vi "tale of three indices.vi"(7 "selector":T2, 11 "tale of three indices -- int -- control":T1={"left"=0, "center"=0, "right"=0, "right most"=0, "left most"=0, "window"=0, "max win factor"=2, "max win"=2, "min win"=2}) -> (0 "no success ?":bool, 1 "at right end?":bool, 3 "tale of three indices -- int -- control out":T1={"left"=0, "center"=0, "right"=0, "right most"=0, "left most"=0, "window"=0, "max win factor"=2, "max win"=2, "min win"=2}, 5 "selector out":T2)   [LabVIEW 2018]
uses:
  tale of three indices -- int -- control.ctl
  tale of three indices -- selector -- control.ctl
  stack action -- control.ctl
  tale of three indices --state.ctl
  Q - not nan -- integer.vi
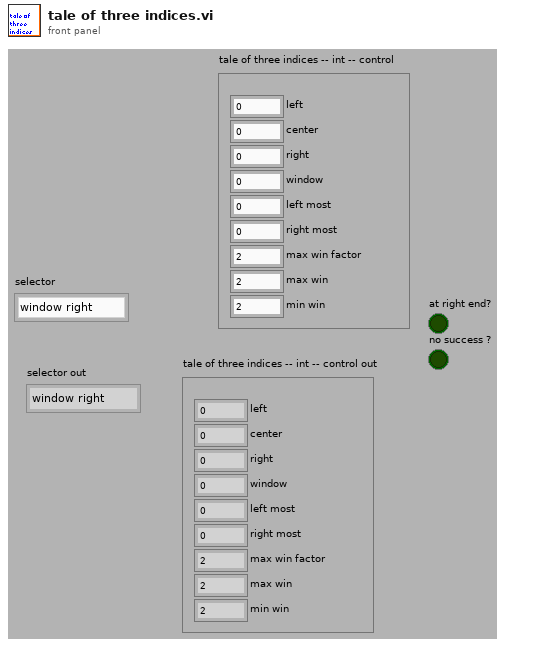
[diagram p1: front panel]
types:
  T1 = typedef "tale of three indices -- int -- control.ctl" = cluster{"left":i32, "center":i32, "right":i32, "right most":i32, "left most":i32, "window":i32, "max win factor":i32, "max win":i32, "min win":i32}
  T2 = typedef "tale of three indices -- selector -- control.ctl" = enum16{"window right", "window left", "balance", "shrink", "grow", "do nothing", "reset", "center right", "center left", "all left", "all right", "right wing shrink", "left wing shrink", "left wing grow", "right wing grow", "skew left", "skew right", "check"}
  T3 = typedef "stack action -- control.ctl" = enum16{"push", "pop", "check", "init"}
  T4 = typedef "tale of three indices --state.ctl" = enum16{"OK", "window stuck at left", "window stuck at right", "left wing shrink - able", "right wing shrink- able", "left wing broaden - able", "window right - able", "right wing broaden - able", "window left - able", "broaden - able", "shrink - able", "center right - able", "center left - able", "balance state"}
  T5 = enum16{"not a number", "above", "in range", "below"}
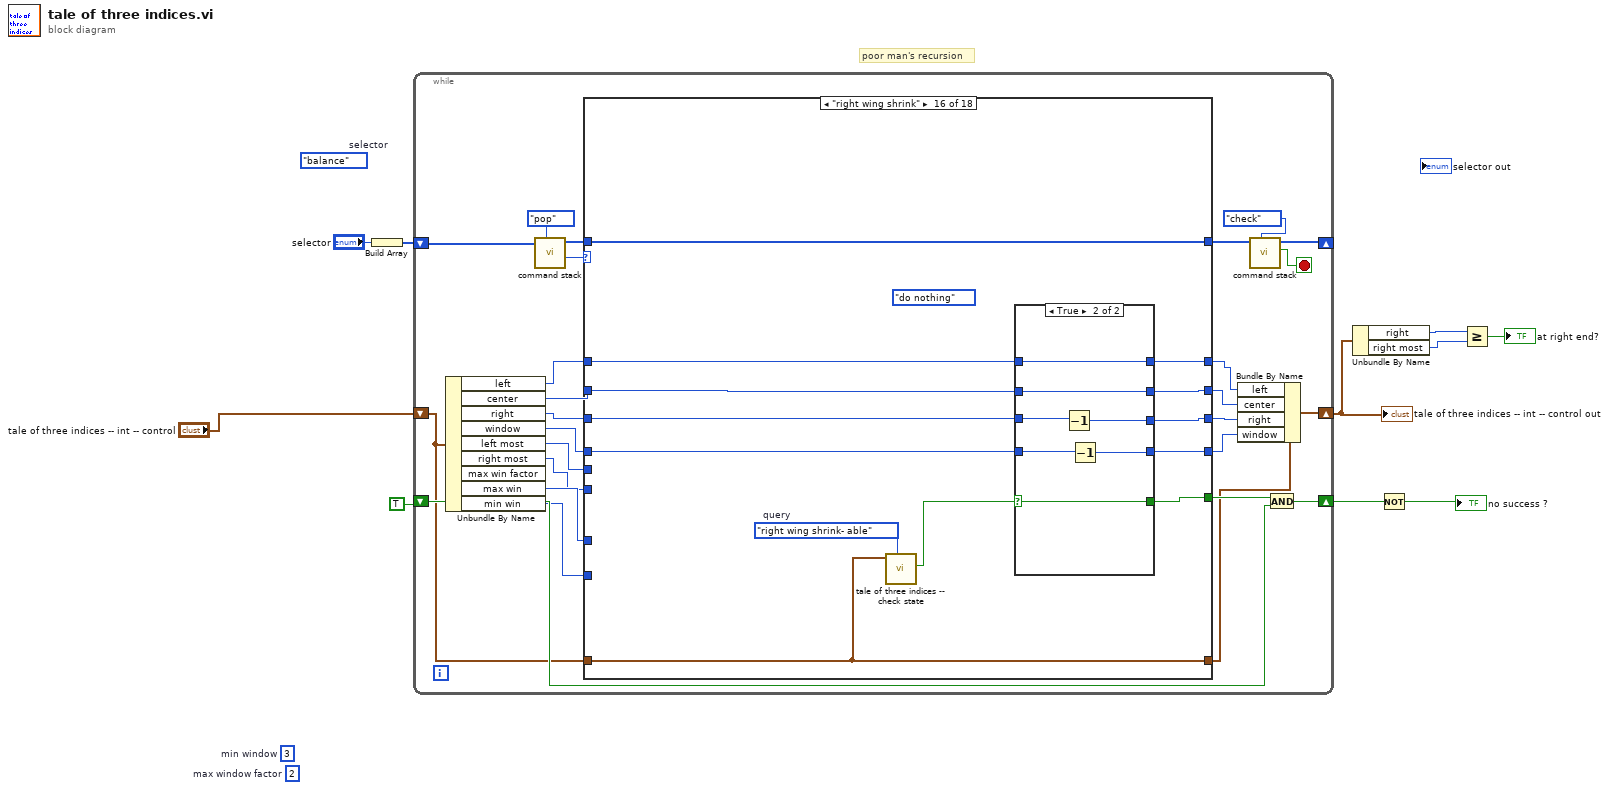
[diagram p0: block diagram]
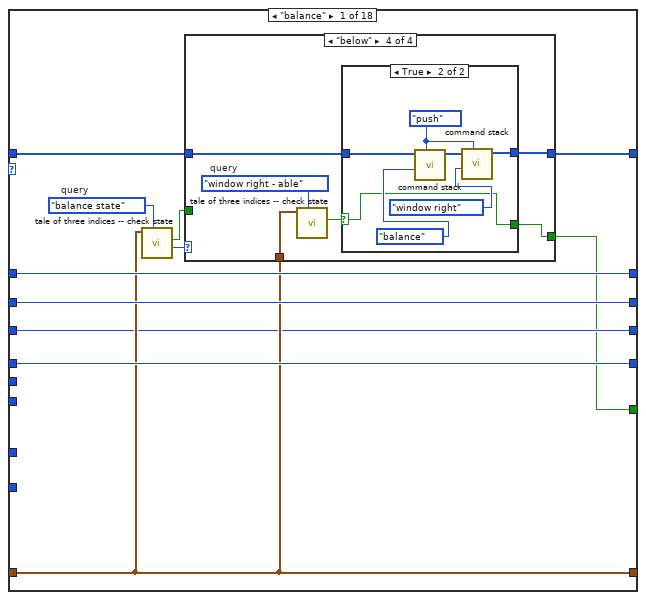
[diagram p2: hidden frame]
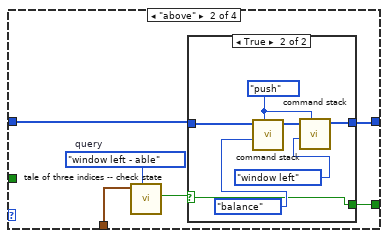
[diagram p4: hidden frame]
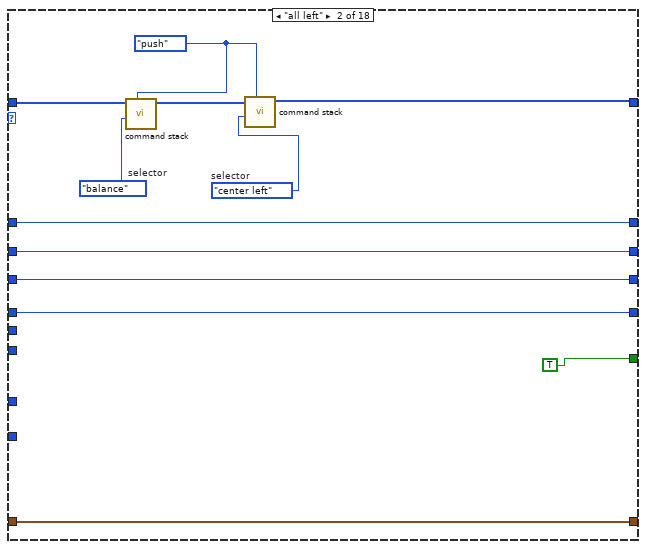
[diagram p8: hidden frame]
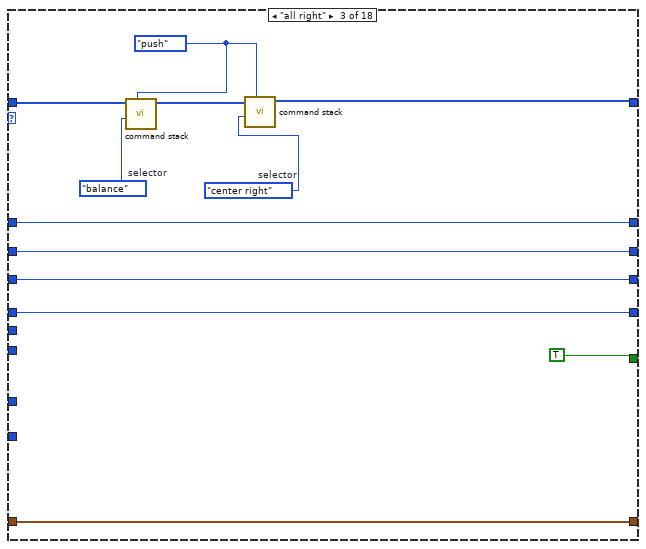
[diagram p9: hidden frame]
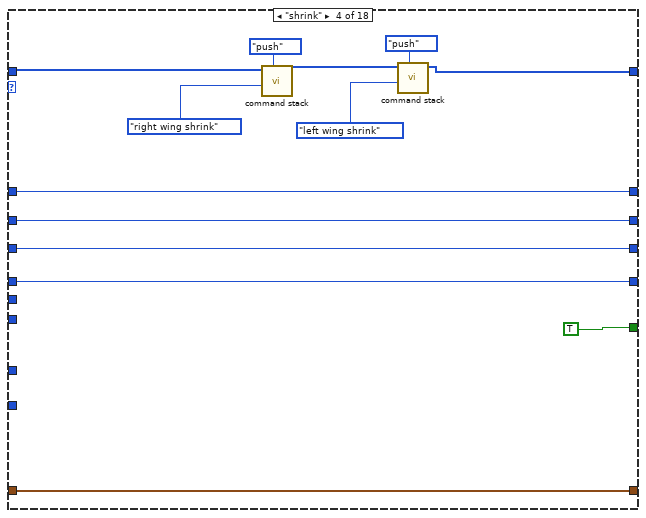
[diagram p10: hidden frame]
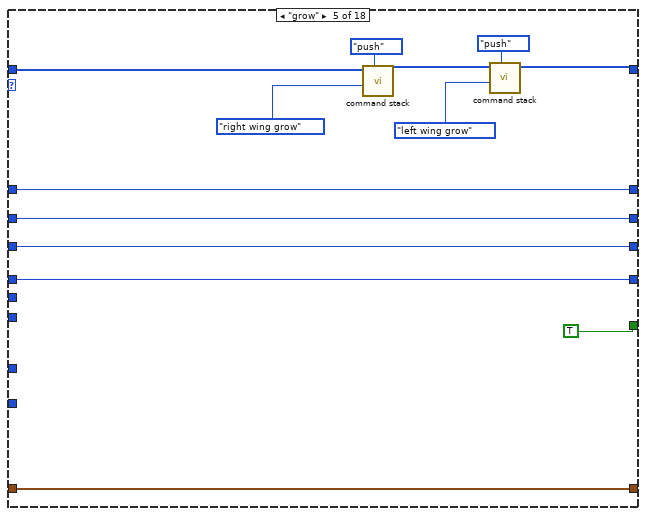
[diagram p11: hidden frame]
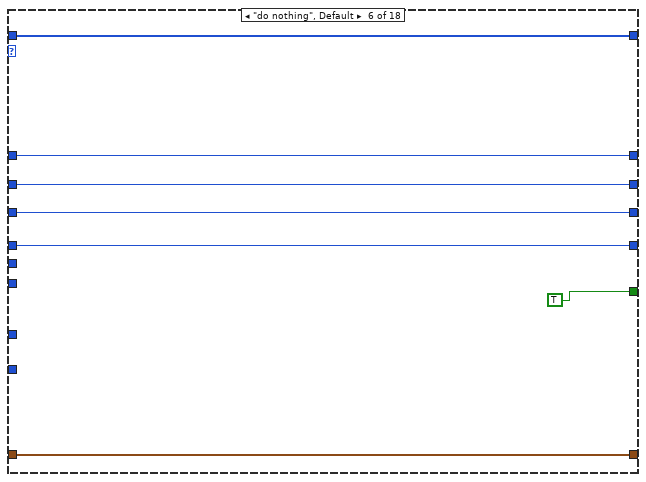
[diagram p12: hidden frame]
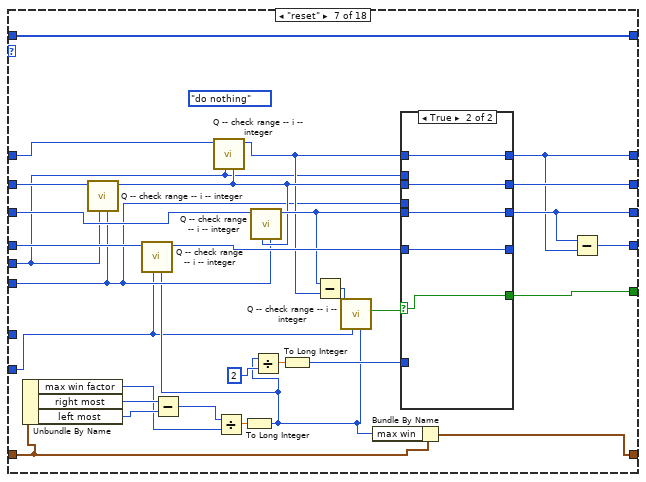
[diagram p13: hidden frame]
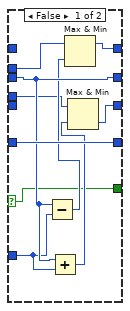
[diagram p14: hidden frame]
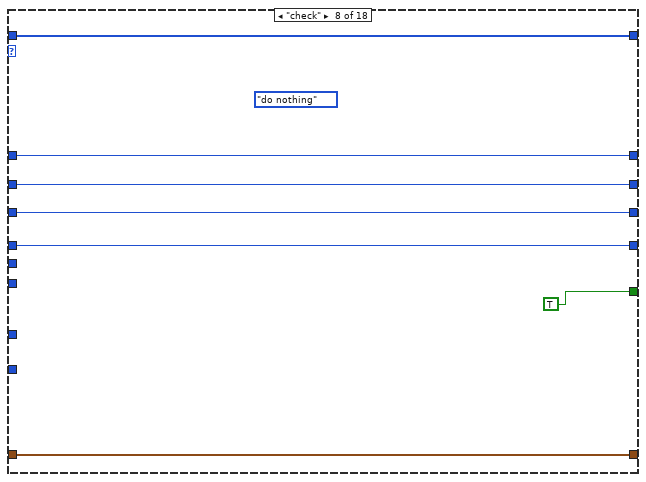
[diagram p15: hidden frame]
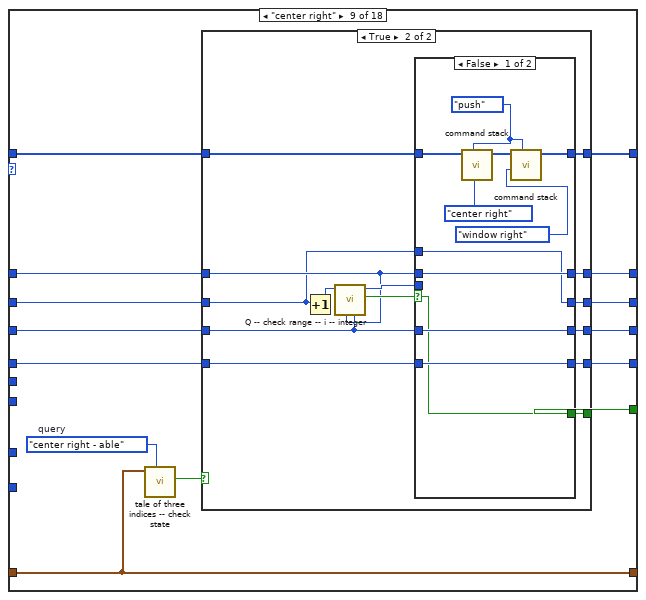
[diagram p16: hidden frame]
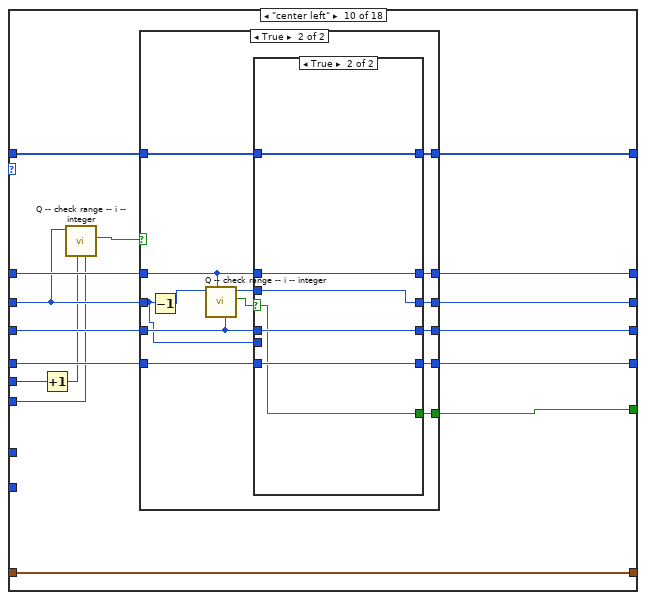
[diagram p19: hidden frame]
diagram:
  (unwired) 2  # max window factor
  (unwired) tale_of_three_indices_--_selector_--_control."balance"  # selector
  (unwired) 3  # min window
  # "poor man's recursion"
  n1 = Build Array("selector") -> (w9:T2[])
  n2 = while {
    shift-right: [w30] -> _
    shift-left: w9 -> [w35]
    shift-right: [w28] -> w6
    shift-left: TRUE -> [w26]
    shift-right: [w24] -> w2
    shift-left: "tale of three indices -- int -- control" -> [w13]
    stop <- w31 stop-if-true
    n3 = Unbundle By Name(w13) -> ("left"=w19:i32, "center"=w18:i32, "right"=w17:i32, "window"=w16:i32, "left most"=w12:i32, "right most"=w11:i32, "max win"=w15:i32, "min win"=w14:i32)  [unwired: 1 out]
    n4 = call "command stack.vi"("action"=stack_action_--_control."pop", "command stack"=w35) -> ("selector out"=w34:T2, "command stack out"=w29:T2[])  [unwired: 7 in, 1 out]
    n5 = case shown="\"right wing shrink\"" w34 {
      tunnel: w19 -> [w42 w86 w98 w116 w122 w137 w165 w189 w203 w256 w296 w327 w335 w357 w383 w408 w435 w454]
      tunnel: [w45 w85 w97 w115 w121 w136 w159 w188 w197 w249 w304 w326 w340 w364 w389 w414 w439 w455] -> w22
      tunnel: w18 -> [w45 w85 w97 w115 w121 w136 w166 w188 w201 w254 w297 w326 w337 w356 w386 w410 w434 w455]
      tunnel: [w42 w86 w98 w116 w122 w137 w149 w189 w198 w250 w303 w327 w339 w363 w388 w413 w440 w454] -> w23
      tunnel: w17 -> [w38 w84 w96 w114 w120 w135 w164 w187 w202 w255 w298 w325 w329 w355 w384 w412 w433 w456]
      tunnel: w11 -> [_ _ _ _ _ _ w152 _ _ w243 _ _ _ _ _ _ _ _]
      tunnel: [w38 w84 w96 w114 w120 w135 w150 w187 w196 w248 w305 w325 w330 w365 w390 w415 w438 w456] -> w21
      tunnel: [w46 w83 w95 w113 w119 w134 w151 w186 w195 w247 w306 w324 w341 w366 w391 w416 w432 w457] -> w20
      tunnel: w16 -> [w46 w83 w95 w113 w119 w134 w167 w186 w194 w246 w295 w324 w334 w354 w382 w407 w431 w457]
      tunnel: w12 -> [_ _ _ _ _ _ w153 _ _ w245 _ _ _ _ _ _ _ _]
      tunnel: w15 -> [_ _ _ _ _ _ _ _ _ _ _ _ _ _ _ _ _ _]
      tunnel: [w43 w90 w102 w108 w123 w133 w148 w185 w200 w252 w302 w320 w338 w362 w387 w411 w441 w460] -> w30
      tunnel: w29 -> [w44 w92 w104 w107 w124 w133 w148 w185 w199 w251 w302 w321 w338 w362 w387 w411 w441 w461]
      tunnel: w14 -> [_ _ _ _ _ _ w138 _ _ _ _ _ _ _ _ _ _ _]
      tunnel: [w37 TRUE TRUE TRUE TRUE TRUE w147 TRUE w193 w242 w301 TRUE w336 w361 w385 w409 w437 TRUE] -> w27
      tunnel: [w39 w82 w94 w117 w130 w132 w140 w184 w191 w241 w299 w328 w333 w358 w380 w404 w429 w463] -> w25
      tunnel: w13 -> [w39 w82 w94 w117 w130 w132 w141 w184 w191 w241 w299 w328 w333 w358 w380 w404 w429 w463]
      frame "balance" {
        w41 = tale_of_three_indices_--state."balance state"  # query
        n6 = call "tale of three indices -- check state.vi"("query"=w41, "tale of three indices"=w39) -> ("balance state"=w40:T5, "answer"=w36:bool)  [unwired: 8 in]
        n7 = case shown="\"below\"" w40 {
          tunnel: w44 -> [w48 w54 w65 w71]
          tunnel: [w48 w53 w65 w70] -> w43
          tunnel: w39 -> [_ w51 _ w68]
          tunnel: [w47 w49 w64 w66] -> w37
          tunnel: w36 -> [w47 _ w64 _]
          frame "not a number", Default {
          }
          frame "above" {
            w50 = tale_of_three_indices_--state."window left - able"  # query
            n8 = call "tale of three indices -- check state.vi"("query"=w50, "tale of three indices"=w51) -> ("answer"=w52:bool)  [unwired: 8 in, 1 out]
            n9 = case shown="True" w52 {
              selector: w52 -> [w55 w57]
              tunnel: w54 -> [w56 w61]
              tunnel: [w56 w60] -> w53
              tunnel: [w55 w57] -> w49
              frame False {
              }
              frame True {
                w63 = stack_action_--_control."push" ("action")
                n10 = call "command stack.vi"("action"=w63, "selector"=tale_of_three_indices_--_selector_--_control."balance" ("selector out"), "command stack"=w61) -> ("command stack out"=w62:T2[])  [unwired: 6 in, 2 out]
                n11 = call "command stack.vi"("action"=w63, "selector"=tale_of_three_indices_--_selector_--_control."window left" ("selector out"), "command stack"=w62) -> ("command stack out"=w60:T2[])  [unwired: 6 in, 2 out]
              }
            }
          }
          frame "in range" {
          }
          frame "below" {
            w69 = tale_of_three_indices_--state."window right - able"  # query
            n12 = call "tale of three indices -- check state.vi"("query"=w69, "tale of three indices"=w68) -> ("answer"=w67:bool)  [unwired: 8 in, 1 out]
            n13 = case shown="True" w67 {
              selector: w67 -> [w72 w74]
              tunnel: w71 -> [w73 w78]
              tunnel: [w73 w77] -> w70
              tunnel: [w72 w74] -> w66
              frame False {
              }
              frame True {
                w80 = stack_action_--_control."push" ("action")
                n14 = call "command stack.vi"("action"=w80, "selector"=tale_of_three_indices_--_selector_--_control."balance" ("selector out"), "command stack"=w78) -> ("command stack out"=w79:T2[])  [unwired: 6 in, 2 out]
                n15 = call "command stack.vi"("action"=w80, "selector"=tale_of_three_indices_--_selector_--_control."window right" ("selector out"), "command stack"=w79) -> ("command stack out"=w77:T2[])  [unwired: 6 in, 2 out]
              }
            }
          }
        }
      }
      frame "all left" {
        w87 = tale_of_three_indices_--_selector_--_control."center left"  # selector
        w88 = tale_of_three_indices_--_selector_--_control."balance"  # selector
        w89 = stack_action_--_control."push" ("action")
        n16 = call "command stack.vi"("action"=w89, "selector"=w88, "command stack"=w92) -> ("command stack out"=w91:T2[])  [unwired: 6 in, 2 out]
        n17 = call "command stack.vi"("action"=w89, "selector"=w87, "command stack"=w91) -> ("command stack out"=w90:T2[])  [unwired: 6 in, 2 out]
      }
      frame "all right" {
        w99 = tale_of_three_indices_--_selector_--_control."center right"  # selector
        w100 = tale_of_three_indices_--_selector_--_control."balance"  # selector
        w101 = stack_action_--_control."push" ("action")
        n18 = call "command stack.vi"("action"=w101, "selector"=w100, "command stack"=w104) -> ("command stack out"=w103:T2[])  [unwired: 6 in, 2 out]
        n19 = call "command stack.vi"("action"=w101, "selector"=w99, "command stack"=w103) -> ("command stack out"=w102:T2[])  [unwired: 6 in, 2 out]
      }
      frame "shrink" {
        n20 = call "command stack.vi"("action"=stack_action_--_control."push", "selector"=tale_of_three_indices_--_selector_--_control."right wing shrink" ("selector out"), "command stack"=w107) -> ("command stack out"=w109:T2[])  [unwired: 6 in, 2 out]
        n21 = call "command stack.vi"("action"=stack_action_--_control."push", "selector"=tale_of_three_indices_--_selector_--_control."left wing shrink" ("selector out"), "command stack"=w109) -> ("command stack out"=w108:T2[])  [unwired: 6 in, 2 out]
      }
      frame "grow" {
        n22 = call "command stack.vi"("action"=stack_action_--_control."push", "selector"=tale_of_three_indices_--_selector_--_control."right wing grow" ("selector out"), "command stack"=w124) -> ("command stack out"=w126:T2[])  [unwired: 6 in, 2 out]
        n23 = call "command stack.vi"("action"=stack_action_--_control."push", "selector"=tale_of_three_indices_--_selector_--_control."left wing grow" ("selector out"), "command stack"=w126) -> ("command stack out"=w123:T2[])  [unwired: 6 in, 2 out]
      }
      frame "do nothing", Default {
      }
      frame "reset" {
        (unwired) tale_of_three_indices_--_selector_--_control."do nothing" ("selector out")
        n24 = Unbundle By Name(w141) -> ("max win factor"=w142:i32, "right most"=w144:i32, "left most"=w143:i32)
        n25 = call "Q -- check range -- i -- integer.vi"("upper"=w152, "lower"=w153, "number"=w166) -> ("number in range"=w158:i32)  [unwired: 6 in, 2 out]
        n26 = Subtract(x=w144, y=w143) -> (x-y=w145:i32)
        n27 = call "Q -- check range -- i -- integer.vi"("upper"=w158, "lower"=w153, "number"=w165) -> ("number in range"=w157:i32)  [unwired: 6 in, 2 out]
        n28 = Divide(x=w145, y=w142) -> (x/y=w146:dbl)
        n29 = To Long Integer(number=w146) -> (32bit integer=w139:i32)
        n30 = call "Q -- check range -- i -- integer.vi"("upper"=w139, "lower"=w138, "number"=w167) -> ("number in range"=w161:i32)  [unwired: 6 in, 2 out]
        n31 = call "Q -- check range -- i -- integer.vi"("upper"=w152, "lower"=w158, "number"=w164) -> ("number in range"=w160:i32)  [unwired: 6 in, 2 out]
        n32 = Divide(x=w139, y=2) -> (x/y=w156:dbl)
        n33 = To Long Integer(number=w156) -> (32bit integer=w154:i32)
        n34 = Subtract(x=w160, y=w157) -> (x-y=w163:i32)
        n35 = call "Q -- check range -- i -- integer.vi"("upper"=w139, "lower"=w138, "number"=w163) -> ("in range?"=w162:bool)  [unwired: 6 in, 2 out]
        n36 = Bundle By Name(cluster=w141, "max win"=w139) -> (w140:T1)
        n37 = case shown="True" w162 {
          selector: w162 -> [w168 w178]
          tunnel: [w177 w182] -> _
          tunnel: w161 -> [w177 w182]
          tunnel: [w169 w181] -> w150
          tunnel: w160 -> [_ w181]
          tunnel: [w176 w180] -> w159
          tunnel: w158 -> [w176 w180]
          tunnel: [w172 w179] -> w149
          tunnel: w157 -> [_ w179]
          tunnel: w154 -> [w175 _]
          tunnel: w153 -> [w173 _]
          tunnel: w152 -> [w170 _]
          tunnel: [w168 w178] -> w147
          frame False {
            n38 = Subtract(x=w176, y=w175) -> (x-y=w174:i32)
            n39 = Add(x=w176, y=w175) -> (x+y=w171:i32)
            n40 = Max & Min(x=w173, y=w174) -> (max(x,y)=w172:i32)  [unwired: 1 out]
            n41 = Max & Min(x=w170, y=w171) -> (min(x,y)=w169:i32)  [unwired: 1 out]
          }
          frame True {
          }
        }
        n42 = Subtract(x=w150, y=w149) -> (x-y=w151:i32)
      }
      frame "check" {
        (unwired) tale_of_three_indices_--_selector_--_control."do nothing" ("selector out")
      }
      frame "center right" {
        w192 = tale_of_three_indices_--state."center right - able"  # query
        n43 = call "tale of three indices -- check state.vi"("query"=w192, "tale of three indices"=w191) -> ("answer"=w190:bool)  [unwired: 8 in, 1 out]
        n44 = case shown="True" w190 {
          selector: w190 -> [w204 _]
          tunnel: w203 -> [w208 w218]
          tunnel: w202 -> [w206 w216]
          tunnel: w201 -> [w207 w211]
          tunnel: [w209 w212] -> w200
          tunnel: w199 -> [w209 w213]
          tunnel: [w208 w219] -> w198
          tunnel: [w207 w221] -> w197
          tunnel: [w206 w217] -> w196
          tunnel: [w205 w215] -> w195
          tunnel: w194 -> [w205 w214]
          tunnel: [w204 w210] -> w193
          frame False {
          }
          frame True {
            n45 = Increment(x=w211) -> (x+1=w223:i32)
            n46 = call "Q -- check range -- i -- integer.vi"("upper"=w216, "lower"=w218, "number"=w223) -> ("in range?"=w222:bool, "number in range"=w220:i32)  [unwired: 6 in, 1 out]
            n47 = case shown="False" w222 {
              selector: w222 -> [w224 w235]
              tunnel: [w227 w240] -> w221
              tunnel: w220 -> [_ w240]
              tunnel: [w228 w239] -> w219
              tunnel: w218 -> [w228 w239]
              tunnel: [w226 w238] -> w217
              tunnel: w216 -> [w226 w238]
              tunnel: [w225 w237] -> w215
              tunnel: w214 -> [w225 w237]
              tunnel: w213 -> [w234 w236]
              tunnel: [w232 w236] -> w212
              tunnel: w211 -> [w227 _]
              tunnel: [w224 w235] -> w210
              frame False {
                w231 = stack_action_--_control."push" ("action")
                n48 = call "command stack.vi"("action"=w231, "selector"=tale_of_three_indices_--_selector_--_control."center right", "command stack"=w234) -> ("command stack out"=w233:T2[])  [unwired: 6 in, 2 out]
                n49 = call "command stack.vi"("action"=w231, "selector"=tale_of_three_indices_--_selector_--_control."window right", "command stack"=w233) -> ("command stack out"=w232:T2[])  [unwired: 6 in, 2 out]
              }
              frame True {
              }
            }
          }
        }
      }
      frame "center left" {
        n50 = Increment(x=w245) -> (x+1=w244:i32)
        n51 = call "Q -- check range -- i -- integer.vi"("upper"=w243, "lower"=w244, "number"=w254) -> ("in range?"=w253:bool)  [unwired: 6 in, 2 out]
        n52 = case shown="True" w253 {
          selector: w253 -> [w257 _]
          tunnel: w256 -> [w261 w271]
          tunnel: w255 -> [w259 w269]
          tunnel: w254 -> [w260 w264]
          tunnel: [w262 w265] -> w252
          tunnel: w251 -> [w262 w266]
          tunnel: [w261 w272] -> w250
          tunnel: [w260 w274] -> w249
          tunnel: [w259 w270] -> w248
          tunnel: [w258 w268] -> w247
          tunnel: w246 -> [w258 w267]
          tunnel: [w257 w263] -> w242
          frame False {
          }
          frame True {
            n53 = Decrement(x=w264) -> (x-1=w276:i32)
            n54 = call "Q -- check range -- i -- integer.vi"("upper"=w269, "lower"=w271, "number"=w276) -> ("in range?"=w275:bool, "number in range"=w273:i32)  [unwired: 6 in, 1 out]
            n55 = case shown="True" w275 {
              selector: w275 -> [w277 w288]
              tunnel: [w280 w293] -> w274
              tunnel: w273 -> [_ w293]
              tunnel: [w281 w292] -> w272
              tunnel: w271 -> [w281 w292]
              tunnel: [w279 w291] -> w270
              tunnel: w269 -> [w279 w291]
              tunnel: [w278 w290] -> w268
              tunnel: w267 -> [w278 w290]
              tunnel: w266 -> [w287 w289]
              tunnel: [w285 w289] -> w265
              tunnel: w264 -> [w280 _]
              tunnel: [w277 w288] -> w263
              frame False {
                w284 = stack_action_--_control."push" ("action")
                n56 = call "command stack.vi"("action"=w284, "selector"=tale_of_three_indices_--_selector_--_control."center left", "command stack"=w287) -> ("command stack out"=w286:T2[])  [unwired: 6 in, 2 out]
                n57 = call "command stack.vi"("action"=w284, "selector"=tale_of_three_indices_--_selector_--_control."window left", "command stack"=w286) -> ("command stack out"=w285:T2[])  [unwired: 6 in, 2 out]
              }
              frame True {
              }
            }
          }
        }
      }
      frame "window left" {
        w300 = tale_of_three_indices_--state."window left - able"  # query
        n58 = call "tale of three indices -- check state.vi"("query"=w300, "tale of three indices"=w299) -> ("answer"=w294:bool)  [unwired: 8 in, 1 out]
        n59 = case shown="True" w294 {
          selector: w294 -> [w309 w316]
          tunnel: [w310 w317] -> w306
          tunnel: [w308 w314] -> w305
          tunnel: w298 -> [w308 w315]
          tunnel: [w311 w318] -> w304
          tunnel: w297 -> [w311 w318]
          tunnel: [w307 w312] -> w303
          tunnel: w296 -> [w307 w313]
          tunnel: w295 -> [w310 w317]
          tunnel: [w309 w316] -> w301
          frame False {
          }
          frame True {
            n60 = Decrement(x=w313) -> (x-1=w312:i32)
            n61 = Decrement(x=w315) -> (x-1=w314:i32)
          }
        }
      }
      frame "skew left" {
        n62 = call "command stack.vi"("action"=stack_action_--_control."push", "selector"=tale_of_three_indices_--_selector_--_control."window left", "command stack"=w321) -> ("command stack out"=w320:T2[])  [unwired: 6 in, 2 out]
      }
      frame "right wing grow" {
        w332 = tale_of_three_indices_--state."right wing broaden - able"  # query
        (unwired) tale_of_three_indices_--_selector_--_control."do nothing" ("selector out")
        n63 = call "tale of three indices -- check state.vi"("query"=w332, "tale of three indices"=w333) -> ("answer"=w331:bool)  [unwired: 8 in, 1 out]
        n64 = case shown="True" w331 {
          selector: w331 -> [w344 w351]
          tunnel: [w345 w349] -> w341
          tunnel: [w346 w353] -> w340
          tunnel: w337 -> [w346 w353]
          tunnel: [w343 w352] -> w339
          tunnel: w335 -> [w343 w352]
          tunnel: w334 -> [w345 w350]
          tunnel: [w344 w351] -> w336
          tunnel: [w342 w347] -> w330
          tunnel: w329 -> [w342 w348]
          frame False {
          }
          frame True {
            n65 = Increment(x=w348) -> (x+1=w347:i32)
            n66 = Increment(x=w350) -> (x+1=w349:i32)
          }
        }
      }
      frame "left wing grow" {
        w360 = tale_of_three_indices_--state."left wing broaden - able"  # query
        (unwired) tale_of_three_indices_--_selector_--_control."do nothing" ("selector out")
        n67 = call "tale of three indices -- check state.vi"("query"=w360, "tale of three indices"=w358) -> ("answer"=w359:bool)  [unwired: 8 in, 1 out]
        n68 = case shown="True" w359 {
          selector: w359 -> [w369 w376]
          tunnel: [w370 w374] -> w366
          tunnel: [w368 w378] -> w365
          tunnel: w355 -> [w368 w378]
          tunnel: [w371 w377] -> w364
          tunnel: w356 -> [w371 w377]
          tunnel: [w367 w372] -> w363
          tunnel: w357 -> [w367 w373]
          tunnel: w354 -> [w370 w375]
          tunnel: [w369 w376] -> w361
          frame False {
          }
          frame True {
            n69 = Increment(x=w375) -> (x+1=w374:i32)
            n70 = Decrement(x=w373) -> (x-1=w372:i32)
          }
        }
      }
      frame "left wing shrink" {
        w381 = tale_of_three_indices_--state."left wing shrink - able"  # query
        (unwired) tale_of_three_indices_--_selector_--_control."do nothing" ("selector out")
        n71 = call "tale of three indices -- check state.vi"("query"=w381, "tale of three indices"=w380) -> ("answer"=w379:bool)  [unwired: 8 in, 1 out]
        n72 = case shown="True" w379 {
          selector: w379 -> [w394 w401]
          tunnel: [w395 w399] -> w391
          tunnel: [w393 w403] -> w390
          tunnel: w384 -> [w393 w403]
          tunnel: [w396 w402] -> w389
          tunnel: w386 -> [w396 w402]
          tunnel: [w392 w397] -> w388
          tunnel: w383 -> [w392 w398]
          tunnel: w382 -> [w395 w400]
          tunnel: [w394 w401] -> w385
          frame False {
          }
          frame True {
            n73 = Increment(x=w398) -> (x+1=w397:i32)
            n74 = Decrement(x=w400) -> (x-1=w399:i32)
          }
        }
      }
      frame "right wing shrink" {
        w406 = tale_of_three_indices_--state."right wing shrink- able"  # query
        (unwired) tale_of_three_indices_--_selector_--_control."do nothing" ("selector out")
        n75 = call "tale of three indices -- check state.vi"("query"=w406, "tale of three indices"=w404) -> ("answer"=w405:bool)  [unwired: 8 in, 1 out]
        n76 = case shown="True" w405 {
          selector: w405 -> [w418 w426]
          tunnel: [w420 w424] -> w416
          tunnel: [w419 w422] -> w415
          tunnel: [w421 w428] -> w414
          tunnel: w410 -> [w421 w428]
          tunnel: [w417 w427] -> w413
          tunnel: w408 -> [w417 w427]
          tunnel: w407 -> [w420 w425]
          tunnel: w412 -> [w419 w423]
          tunnel: [w418 w426] -> w409
          frame False {
          }
          frame True {
            n77 = Decrement(x=w423) -> (x-1=w422:i32)
            n78 = Decrement(x=w425) -> (x-1=w424:i32)
          }
        }
      }
      frame "window right" {
        w436 = tale_of_three_indices_--state."window right - able"  # query
        (unwired) TRUE
        (unwired) tale_of_three_indices_--_selector_--_control."do nothing" ("selector out")
        n79 = call "tale of three indices -- check state.vi"("query"=w436, "tale of three indices"=w429) -> ("answer"=w430:bool)  [unwired: 8 in, 1 out]
        n80 = case shown="True" w430 {
          selector: w430 -> [w445 w451]
          tunnel: [w442 w452] -> w432
          tunnel: [w443 w449] -> w438
          tunnel: w433 -> [w443 w450]
          tunnel: [w446 w453] -> w439
          tunnel: w434 -> [w446 w453]
          tunnel: [w444 w448] -> w440
          tunnel: w435 -> [w444 w447]
          tunnel: w431 -> [w442 w452]
          tunnel: [w445 w451] -> w437
          frame False {
          }
          frame True {
            n81 = Increment(x=w450) -> (x+1=w449:i32)
            n82 = Increment(x=w447) -> (x+1=w448:i32)
          }
        }
      }
      frame "skew right" {
        n83 = call "command stack.vi"("action"=stack_action_--_control."push", "selector"=tale_of_three_indices_--_selector_--_control."window right", "command stack"=w461) -> ("command stack out"=w460:T2[])  [unwired: 6 in, 2 out]
      }
    }
    n84 = Bundle By Name(cluster=w25, "left"=w23, "center"=w22, "right"=w21, "window"=w20) -> (w24:T1)
    n85 = call "command stack.vi"("action"=stack_action_--_control."check", "command stack"=w30) -> ("stack is empty ?"=w31:bool)  [unwired: 7 in, 2 out]
    n86 = And(x=w27, y=w26) -> (x .and. y?=w28:bool)
  }
  "tale of three indices -- int -- control out" <- w2
  n87 = Unbundle By Name(w2) -> ("right"=w1:i32, "right most"=w8:i32)
  n88 = Not(x=w6) -> (.not. x?=→"no success ?":bool)
  n89 = Greater Or Equal?(x=w1, y=w8) -> (x >= y?=→"at right end?":bool)
